vi "ToXML.vi"(5 "TestCase":refnum<class "TestCase.lvclass">, 6 "error in":errorcluster, 9 "DOM document":refnum<k20>) -> (0 "error out":errorcluster, 3 "DOM document out":refnum<k20>, 4 "TestCase element":refnum<k20>)   [LabVIEW 2014, in "TestCase.lvclass"]
uses:
  TestCase.lvclass
  TestCase.lvclass/TestCase.ctl
  <resource>/objmgr/DOMUserDefRef.rc
  <vilib>/xml/NI_XML.lvlib
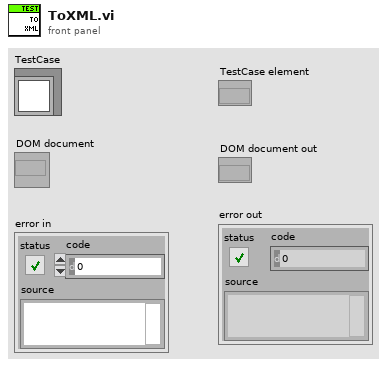
[diagram p1: front panel]
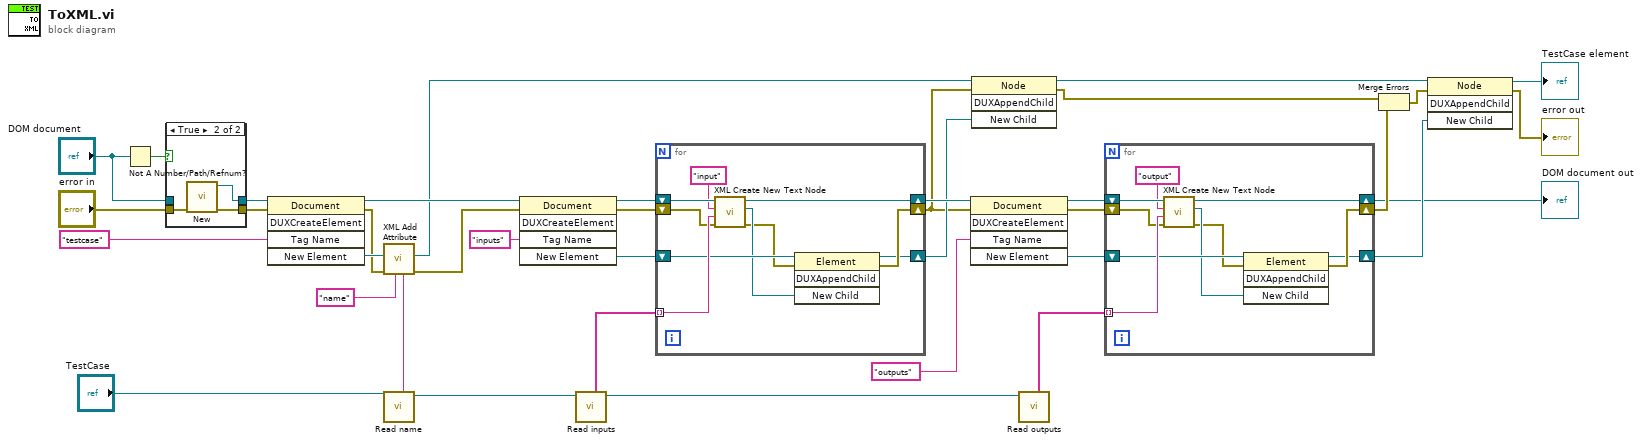
[diagram p0: block diagram]
diagram:
  n1 = Not A Number/Path/Refnum?(number/path/refnum="DOM document") -> (NaN/Path/Refnum?=w6:bool)
  n2 = case shown="True" w6 {
    tunnel: "error in" -> [w39 w42]
    tunnel: "DOM document" -> [w38 _]
    tunnel: [w39 w41] -> w3
    tunnel: [w38 w40] -> w2
    frame False {
    }
    frame True {
      n3 = call <vilib>:"New.vi"("error in (no error)"=w42) -> ("error out"=w41:errorcluster, "DOM document out"=w40:refnum<k20>)  [unwired: 7 in]
    }
  }
  n4 = invoke class="Document" method="DUXCreateElement"(reference=w2, error in=w3, "Tag Name"="testcase") -> (reference out=w27:refnum<k20>, error out=w35:errorcluster, "New Element"=w36:refnum<k20>)  [unwired: 2 in, 2 out]
  n5 = call "Read name.vi"("TestCase in"="TestCase") -> ("TestCase out"=w20:refnum<class "TestCase.lvclass">, "name"=w34:string)  [unwired: 7 in]
  n6 = call "XML Add Attribute.vi"("Value"=w34, "Name"="name", "error in"=w35, "element"=w36) -> ("error out"=w26:errorcluster, "element out"=w17:refnum<k20>)  [unwired: 4 in]
  n7 = invoke class="Document" method="DUXCreateElement"(reference=w27, error in=w26, "Tag Name"="inputs") -> (reference out=w30:refnum<k20>, error out=w29:errorcluster, "New Element"=w31:refnum<k20>)  [unwired: 2 in, 2 out]
  n8 = call "Read inputs.vi"("TestCase in"=w20) -> ("TestCase out"=w19:refnum<class "TestCase.lvclass">, "inputs"=w21:string[])  [unwired: 7 in]
  n9 = for {
    shift-right: [w44] -> w16
    shift-left: w31 -> [w48]
    shift-right: [w43] -> w24
    shift-left: w30 -> [w52]
    shift-right: [w45] -> w15
    shift-left: w29 -> [w49]
    tunnel: w21 -> [w50] mode=indexing
    n10 = call "XML Create New Text Node.vi"("error in (no error)"=w49, "Data"=w50, "Tag Name"="input", "DOM document"=w52) -> ("error out"=w46:errorcluster, "New Element"=w47:refnum<k20>, "DOM document out"=w43:refnum<k20>)  [unwired: 5 in]
    n11 = invoke class="Element" method="DUXAppendChild"(reference=w48, error in=w46, "New Child"=w47) -> (reference out=w44:refnum<k20>, error out=w45:errorcluster)  [unwired: 1 in, 2 out]
  }
  n12 = invoke class="Document" method="DUXCreateElement"(reference=w24, error in=w15, "Tag Name"="outputs") -> (reference out=w23:refnum<k20>, error out=w22:errorcluster, "New Element"=w1:refnum<k20>)  [unwired: 2 in, 2 out]
  n13 = invoke class="Node" method="DUXAppendChild"(reference=w17, error in=w15, "New Child"=w16) -> (reference out=w14:refnum<k20>, error out=w12:errorcluster)  [unwired: 1 in, 2 out]
  n14 = call "Read outputs.vi"("TestCase in"=w19) -> ("outputs"=w18:string[])  [unwired: 7 in, 1 out]
  n15 = for {
    shift-right: [w54] -> w13
    shift-left: w1 -> [w58]
    shift-right: [w53] -> w8
    shift-left: w23 -> [w62]
    shift-right: [w55] -> w10
    shift-left: w22 -> [w59]
    tunnel: w18 -> [w60] mode=indexing
    n16 = call "XML Create New Text Node.vi"("error in (no error)"=w59, "Data"=w60, "Tag Name"="output", "DOM document"=w62) -> ("error out"=w56:errorcluster, "New Element"=w57:refnum<k20>, "DOM document out"=w53:refnum<k20>)  [unwired: 5 in]
    n17 = invoke class="Element" method="DUXAppendChild"(reference=w58, error in=w56, "New Child"=w57) -> (reference out=w54:refnum<k20>, error out=w55:errorcluster)  [unwired: 1 in, 2 out]
  }
  "DOM document out" <- w8
  n18 = Merge Errors(w12, w10) -> (w11:errorcluster)
  n19 = invoke class="Node" method="DUXAppendChild"(reference=w14, error in=w11, "New Child"=w13) -> (reference out=→"TestCase element":refnum<k20>, error out=→"error out":errorcluster)  [unwired: 1 in, 2 out]
